vi "State.enabled.controls.vi"(11 "state":i32) -> (0 "live":T1(ring), 1 "pause":T1(ring), 2 "abort":T1(ring), 3 "start":T1(ring), 4 "stop":T1(ring))   [LabVIEW 2022 SP3]
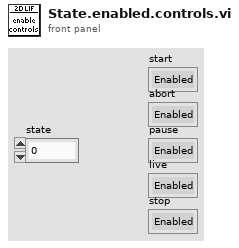
[diagram p1: front panel]
types:
  T1 = enum8{"Enabled", "Disabled", "Disabled and Grayed Out"}
  T2 = enum8{"Enabled", "Disabled", "Disabled and Grayed Out"}[][]
  T3 = enum8{"Enabled", "Disabled", "Disabled and Grayed Out"}[]
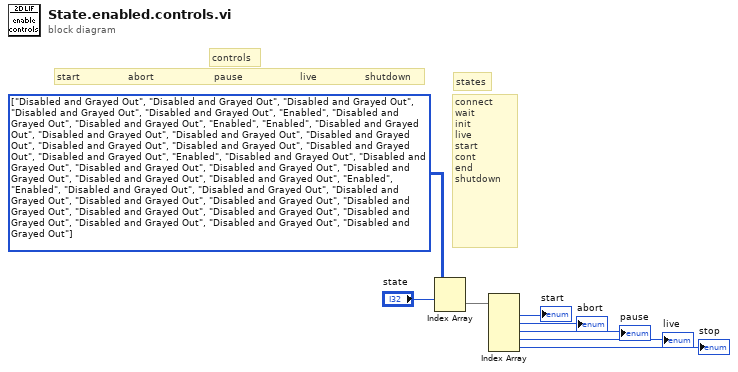
[diagram p0: block diagram]
diagram:
  w8 = T2 [[enum."Disabled and Grayed Out", enum."Disabled and Grayed Out", enum."Disabled and Grayed Out", enum."Disabled and Grayed Out", enum."Disabled and Grayed Out"], [enum."Enabled", enum."Disabled and Grayed Out", enum."Disabled and Grayed Out", enum."Enabled", enum."Enabled"], [enum."Disabled and Grayed Out", enum."Disabled and Grayed Out", enum."Disabled and Grayed Out", enum."Disabled and Grayed Out", enum."Disabled and Grayed Out"], [enum."Disabled and Grayed Out", enum."Disabled and Grayed Out", enum."Disabled and Grayed Out", enum."Enabled", enum."Disabled and Grayed Out"], [enum."Disabled and Grayed Out", enum."Disabled and Grayed Out", enum."Disabled and Grayed Out", enum."Disabled and Grayed Out", enum."Disabled and Grayed Out"], [enum."Disabled and Grayed Out", enum."Enabled", enum."Enabled", enum."Disabled and Grayed Out", enum."Disabled and Grayed Out"], [enum."Disabled and Grayed Out", enum."Disabled and Grayed Out", enum."Disabled and Grayed Out", enum."Disabled and Grayed Out", enum."Disabled and Grayed Out"], [enum."Disabled and Grayed Out", enum."Disabled and Grayed Out", enum."Disabled and Grayed Out", enum."Disabled and Grayed Out", enum."Disabled and Grayed Out"]] items=["Enabled", "Disabled", "Disabled and Grayed Out"]
  # "states"
  # "controls"
  # "connect\nwait\ninit\nlive\nstart\ncont\nend\nshutdown"
  # "start                abort                    pause                   live                shutdown"
  n1 = Index Array(array=w8, index (row)="state") -> (element=w6:T3)  [unwired: 1 in]
  n2 = Index Array(array=w6) -> (element #1=→"start":T1, element #2=→"abort":T1, element #3=→"pause":T1, element #4=→"live":T1, element #5=→"stop":T1)  [unwired: 5 in]
